vi "ADIS16470 Loop Write Config.vi"(8 "error in (no error)":errorcluster, 10 "Calibration Time":T3, 11 "SPIDevRef":T1) -> (0 "error out":errorcluster)   [LabVIEW 2019]
uses:
  Typedef/ADIS16470 Calibration Time.ctl
  <vilib>/Rock Robotics/WPI/SPI/WPI_SPIDevRef.ctl
  <vilib>/Rock Robotics/SystemInterfaces/spilib/spi_bus.ctl
  Typedef/ADIS16470 Register.ctl
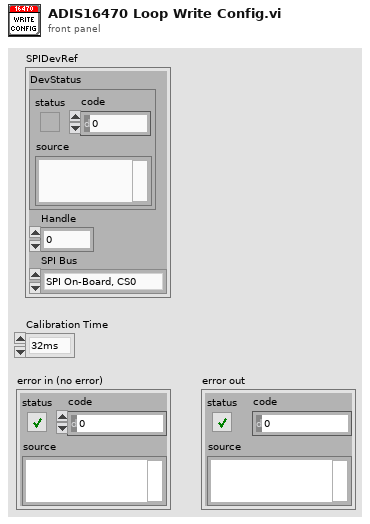
[diagram p1: front panel]
types:
  T1 = typedef "WPI_SPIDevRef.ctl" = cluster{"DevStatus":errorcluster, "Handle":i32, "SPI Bus":T2}
  T2 = typedef "spi_bus.ctl" = enum16{"SPI On-Board, CS0", "SPI On-Board, CS1", "SPI On-Board, CS2", "SPI On-Board, CS3", "SPI MXP", "Invalid"}
  T3 = typedef "ADIS16470 Calibration Time.ctl" = enum16{"32ms", "64ms", "128ms", "256ms", "512ms", "1s", "2s", "4s", "8s", "16s", "32s", "64s"}
  T4 = typedef "ADIS16470 Register.ctl" = u8
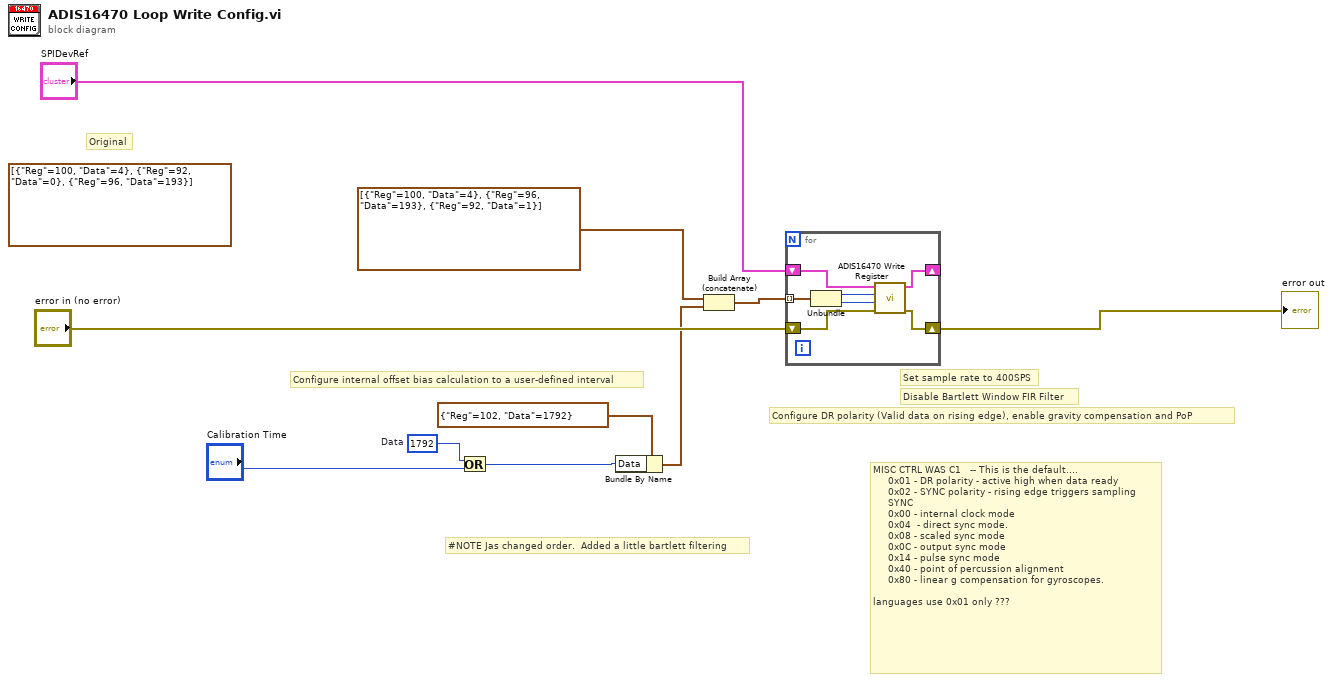
[diagram p0: block diagram]
diagram:
  (unwired) cluster{"Reg":T4, "Data":u16}[] [{"Reg"=100, "Data"=4}, {"Reg"=92, "Data"=0}, {"Reg"=96, "Data"=193}]
  w8 = 1792  # Data
  # "#NOTE Jas changed order.  Added a little bartlett filtering"
  # "Original"
  # "MISC CTRL WAS C1   -- This is the default....\n     0x01 - DR polarity - active high when data ready\n     0x02 - SYNC polarity - rising edge triggers sampling\n     SYNC\n     0x00 - internal clock mode\n     0x04  - direct sync mode.\n     0x08 - scaled sync mode\n     0x0C - output sync mode\n     0x14 - pulse sync mode\n     0x40 - point of percussion alignment\n     0x80 - linear g compensation for gyroscopes.\n\nlanguages use 0x01 only ???"
  # "Set sample rate to 400SPS"
  # "Configure internal offset bias calculation to a user-defined interval"
  # "Configure DR polarity (Valid data on rising edge), enable gravity compensation and PoP"
  # "Disable Bartlett Window FIR Filter"
  n1 = Or(x=w8, y="Calibration Time") -> (x .or. y?=w9:i32)
  n2 = Bundle By Name(cluster=cluster{"Reg":T4, "Data":i32} {"Reg"=102, "Data"=1792}, "Data"=w9) -> (w1:cluster{"Reg":T4, "Data":i32})
  n3 = Build Array (concatenate)(cluster{"Reg":T4, "Data":u16}[] [{"Reg"=100, "Data"=4}, {"Reg"=96, "Data"=193}, {"Reg"=92, "Data"=1}], w1) -> (w7:cluster{"Reg":T4, "Data":i32}[])
  n4 = for {
    tunnel: w7 -> [w11] mode=indexing
    shift-right: [w14] -> w4
    shift-left: "error in (no error)" -> [w13]
    shift-right: [w12] -> _
    shift-left: "SPIDevRef" -> [w15]
    n5 = Unbundle(w11) -> ("Reg"=w17:T4, "Data"=w16:i32)
    n6 = call "ADIS16470 Write Register.vi"("error in (no error)"=w13, "Data"=w16, "Register"=w17, "SPIDevRef in"=w15) -> ("error out"=w14:errorcluster, "SPIDevRef out"=w12:T1)  [unwired: 6 in]
  }
  "error out" <- w4
